vi "sensorTestOutput.vi"() -> ()   [LabVIEW 2018]
panel:
  out "max":dbl
  out "driveAvgFt/s":dbl
  in  "Reset Encoder (Make sure false)":bool
  out "Bound Angle":dbl
  out "climbPoweredIRLeft":bool
  out "climbSkidIRRight":bool
  out "climbPoweredIRRight":bool
  out "lineIRFrontLeft":bool
  out "lineIRFrontRight":bool
  out "lineIRRearLeft":bool
  out "climbSkidIRLeft":bool
  out "cargoYellowIRCVal":bool
  out "lineIRRearRight":bool
  out "driveLeftPositionInch":dbl
  out "driveRightPositionInch":dbl
  out "Button_Y(3)":bool
  out "Button_X(0)":bool
  out "Button_Start(9)":bool
  out "Button_RT(7)":bool
  out "Button_RB(5)":bool
  out "Button_LT(6)":bool
  out "Button_LB(4)":bool
  out "Button_D_Pad_Up(0)":bool
  out "Button_D_Pad_Right(90)":bool
  out "Button_D_Pad_Left(270)":bool
  out "Button_D_Pad_Down(180)":bool
  out "Button_Back(8)":bool
  out "Button_B(2)":bool
  out "Button_A(1)":bool
  out "Axis_Right_Y(3)":dbl
  out "Axis_Right_X(2)":dbl
  out "Axis_Left_Y(1)":dbl
  out "Axis_Left_X(0)":dbl
  out "pitchWind":dbl
  out "yawWind":dbl
  out "driveRightEncoderPosition":i32
  out "driveLeftEncoderPosition":i32
  out "driveIMUYawPitchRoll":cluster{"Yaw":dbl, "Pitch":dbl, "Roll":dbl}
  out "driveFusedHeading":T1
  out "climbRearPosition":i32
  out "climbFrontPosition":i32
  out "rollwind":dbl
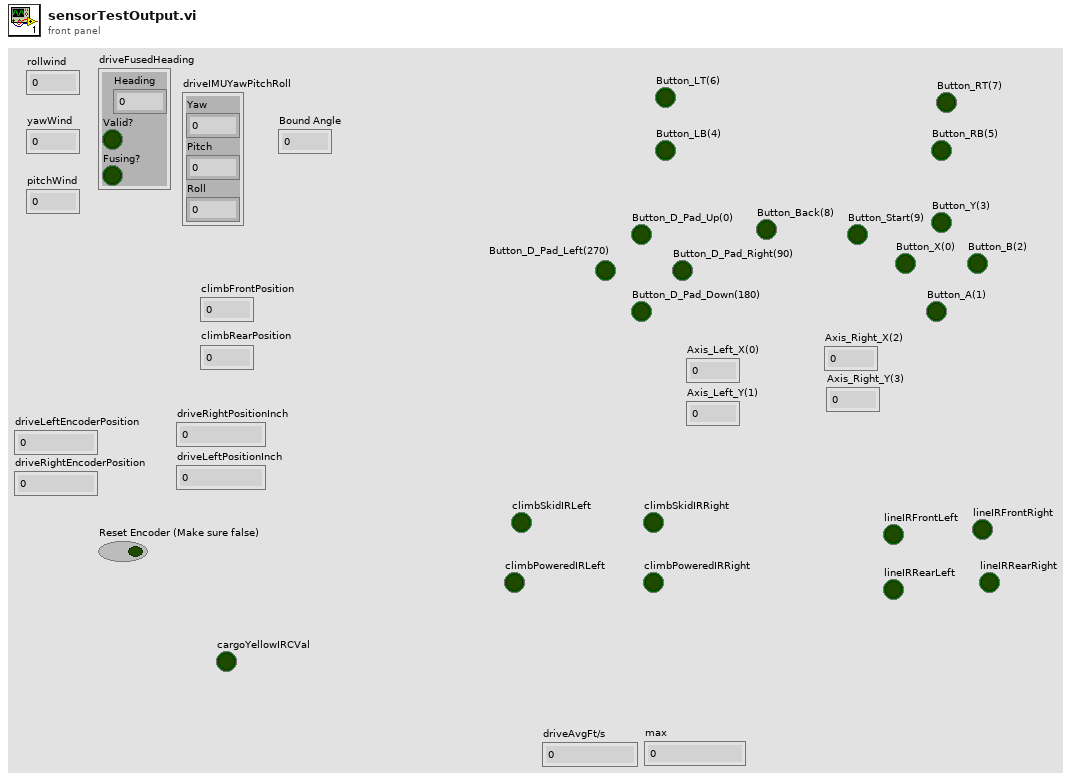
[diagram p1: front panel]
types:
  T1 = cluster{"Heading":dbl, "Valid?":bool, "Fusing?":bool}
  T2 = enum16{"[0, 360]", "[-180, 180]", "[0, 2PI]", "[-PI, PI]"}
  T3 = typedef "WPI_MotorControlDeviceRef.ctl" = cluster{"DeviceStatus":errorcluster, "Type":T4, "PWM":cluster{"PWM Channel":T5, "DeadBand":T6}, "CAN":cluster{"Device Number":u8, "SetOutput VI Ref":variant, "GetOutput VI Ref":variant, "Enable VI Ref":variant, "Disable VI Ref":variant, "Data":variant}, "Invert":bool, "DIO PWM":cluster{"PWM \"Enable\" Channel":T5, "DIOChannel":T7, "PWM Rate":dbl}}
  T4 = typedef "WPI_MotorControlType.ctl" = enum16{"PWM", "CAN", "DIO PWM"}
  T5 = typedef "FPGA_DIOPWMChannel.ctl" = enum8{"PWM 0", "PWM 1", "PWM 2", "PWM 3", "PWM 4", "PWM 5", "PWM 6", "PWM 7", "PWM 8", "PWM 9", "PWM MXP 0", "PWM MXP 1", "PWM MXP 2", "PWM MXP 3", "PWM MXP 4", "PWM MXP 5", "PWM MXP 6", "PWM MXP 7", "PWM MXP 8", "PWM MXP 9", "Invalid"}
  T6 = typedef "WPI_PWMDeadband.ctl" = cluster{"Name":string, "maxPositivePwm":i32, "minPositivePwm":i32, "centerPwm":i32, "maxNegativePwm":i32, "minNegativePwm":i32, "angularRange":u16}
  T7 = typedef "FPGA_DIOChannel.ctl" = enum8{"DIO 0", "DIO 1", "DIO 2", "DIO 3", "DIO 4", "DIO 5", "DIO 6", "DIO 7", "DIO 8", "DIO 9", "DIO MXP 0", "DIO MXP 1", "DIO MXP 2", "DIO MXP 3", "DIO MXP 4", "DIO MXP 5", "DIO MXP 6", "DIO MXP 7", "DIO MXP 8", "DIO MXP 9", "DIO MXP 10", "DIO MXP 11", "DIO MXP 12", "DIO MXP 13", "DIO MXP 14", "DIO MXP 15", "SPI Port CS1", "SPI Port CS2", "SPI Port CS3", "SPI Port MISO", "SPI Port MOSI", "Invalid"}
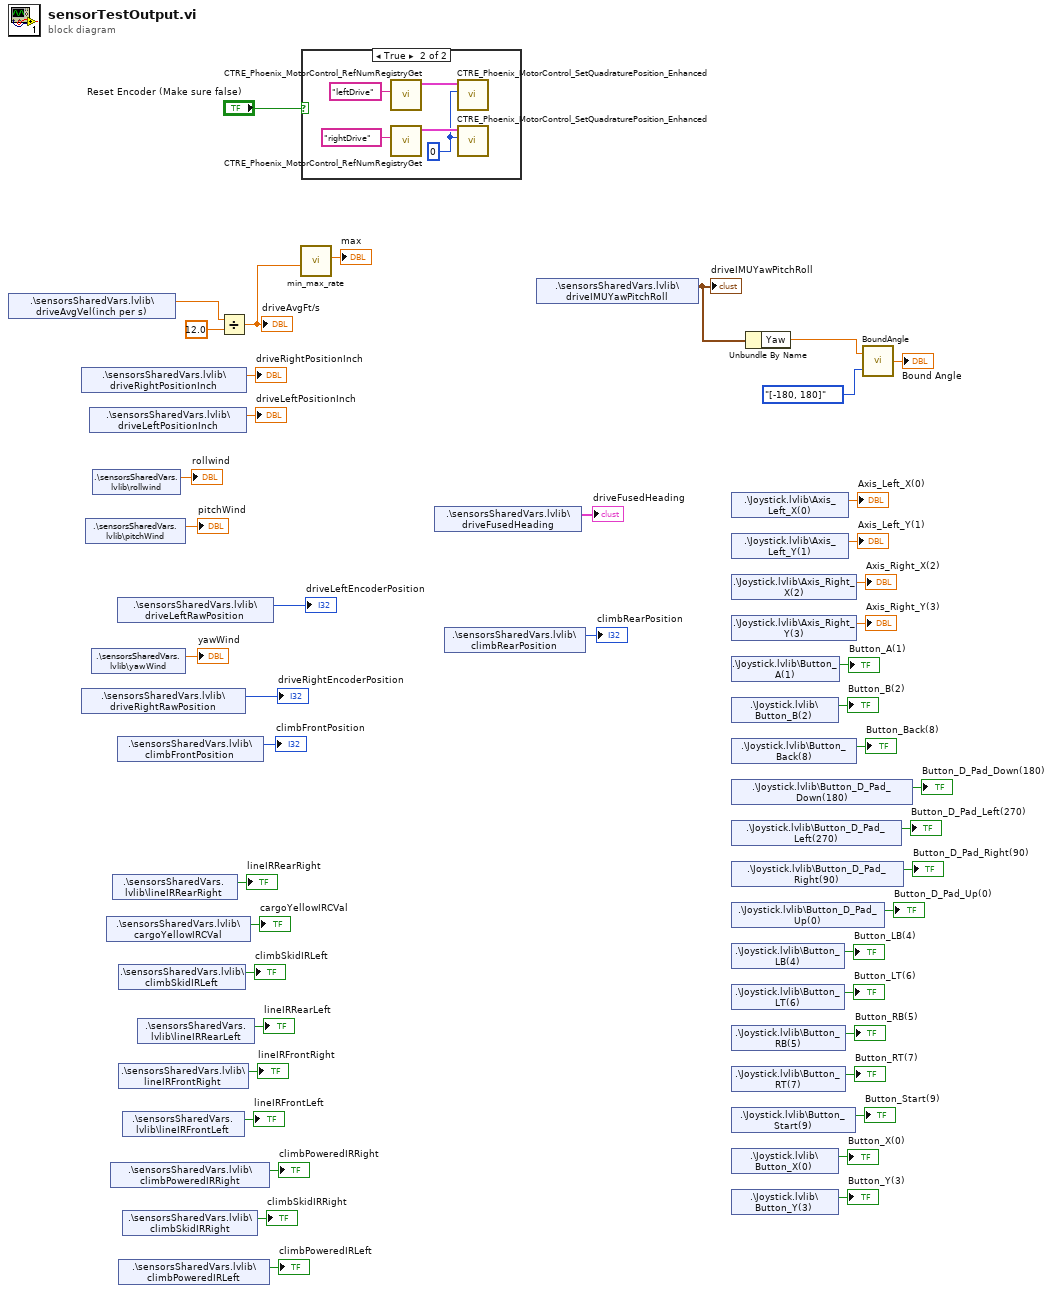
[diagram p0: block diagram]
diagram:
  n1 = shared-variable ".\\sensorsSharedVars.lvlib\\driveAvgVel(inch per s)"() -> (w4:dbl)  [unwired: 1 in, 1 out]
  n2 = shared-variable ".\\sensorsSharedVars.lvlib\\driveRightPositionInch"() -> (→"driveRightPositionInch":dbl)  [unwired: 1 in, 1 out]
  n3 = shared-variable ".\\sensorsSharedVars.lvlib\\driveRightRawPosition"() -> (→"driveRightEncoderPosition":i32)  [unwired: 1 in, 1 out]
  n4 = shared-variable ".\\sensorsSharedVars.lvlib\\pitchWind"() -> (→"pitchWind":dbl)  [unwired: 1 in, 1 out]
  n5 = shared-variable ".\\sensorsSharedVars.lvlib\\driveLeftPositionInch"() -> (→"driveLeftPositionInch":dbl)  [unwired: 1 in, 1 out]
  n6 = shared-variable ".\\sensorsSharedVars.lvlib\\yawWind"() -> (→"yawWind":dbl)  [unwired: 1 in, 1 out]
  n7 = shared-variable ".\\sensorsSharedVars.lvlib\\rollwind"() -> (→"rollwind":dbl)  [unwired: 1 in, 1 out]
  n8 = shared-variable ".\\sensorsSharedVars.lvlib\\cargoYellowIRCVal"() -> (→"cargoYellowIRCVal":bool)  [unwired: 1 in, 1 out]
  n9 = shared-variable ".\\sensorsSharedVars.lvlib\\climbPoweredIRRight"() -> (→"climbPoweredIRRight":bool)  [unwired: 1 in, 1 out]
  n10 = shared-variable ".\\sensorsSharedVars.lvlib\\lineIRRearRight"() -> (→"lineIRRearRight":bool)  [unwired: 1 in, 1 out]
  n11 = shared-variable ".\\sensorsSharedVars.lvlib\\driveLeftRawPosition"() -> (→"driveLeftEncoderPosition":i32)  [unwired: 1 in, 1 out]
  n12 = shared-variable ".\\sensorsSharedVars.lvlib\\climbFrontPosition"() -> (→"climbFrontPosition":i32)  [unwired: 1 in, 1 out]
  n13 = shared-variable ".\\sensorsSharedVars.lvlib\\climbSkidIRLeft"() -> (→"climbSkidIRLeft":bool)  [unwired: 1 in, 1 out]
  n14 = shared-variable ".\\sensorsSharedVars.lvlib\\lineIRFrontRight"() -> (→"lineIRFrontRight":bool)  [unwired: 1 in, 1 out]
  n15 = shared-variable ".\\sensorsSharedVars.lvlib\\climbPoweredIRLeft"() -> (→"climbPoweredIRLeft":bool)  [unwired: 1 in, 1 out]
  n16 = shared-variable ".\\sensorsSharedVars.lvlib\\lineIRFrontLeft"() -> (→"lineIRFrontLeft":bool)  [unwired: 1 in, 1 out]
  n17 = shared-variable ".\\sensorsSharedVars.lvlib\\climbSkidIRRight"() -> (→"climbSkidIRRight":bool)  [unwired: 1 in, 1 out]
  n18 = shared-variable ".\\sensorsSharedVars.lvlib\\lineIRRearLeft"() -> (→"lineIRRearLeft":bool)  [unwired: 1 in, 1 out]
  n19 = Divide(x=w4, y=12.0) -> (x/y=w2:dbl)
  "driveAvgFt/s" <- w2
  n20 = call "min_max_rate.vi"("Rate"=w2) -> ("max"=→"max":dbl)  [unwired: 9 in, 1 out]
  n21 = case shown="True" "Reset Encoder (Make sure false)" {
    frame False {
    }
    frame True {
      w47 = 0 ("New Sensor Position")
      n22 = call <vilib>:"CTRE_Phoenix_MotorControl_RefNumRegistryGet.vi"("refnum name"="leftDrive") -> ("PhoenixMotorControlDevRef"=w49:T3)  [unwired: 9 in, 1 out]
      n23 = call <vilib>:"CTRE_Phoenix_MotorControl_RefNumRegistryGet.vi"("refnum name"="rightDrive") -> ("PhoenixMotorControlDevRef"=w48:T3)  [unwired: 9 in, 1 out]
      n24 = call <vilib>:"CTRE_Phoenix_MotorControl_SetQuadraturePosition_Enhanced.vi"("New Position"=w47, "PhoenixMotorControlDevRef"=w49) -> ()  [unwired: 8 in, 2 out]
      n25 = call <vilib>:"CTRE_Phoenix_MotorControl_SetQuadraturePosition_Enhanced.vi"("New Position"=w47, "PhoenixMotorControlDevRef"=w48) -> ()  [unwired: 8 in, 2 out]
    }
  }
  n26 = shared-variable ".\\sensorsSharedVars.lvlib\\driveFusedHeading"() -> (→"driveFusedHeading":T1)  [unwired: 1 in, 1 out]
  n27 = shared-variable ".\\sensorsSharedVars.lvlib\\climbRearPosition"() -> (→"climbRearPosition":i32)  [unwired: 1 in, 1 out]
  n28 = shared-variable ".\\sensorsSharedVars.lvlib\\driveIMUYawPitchRoll"() -> (w9:cluster{"Yaw":dbl, "Pitch":dbl, "Roll":dbl})  [unwired: 1 in, 1 out]
  "driveIMUYawPitchRoll" <- w9
  n29 = shared-variable ".\\Joystick.lvlib\\Axis_Left_X(0)"() -> (→"Axis_Left_X(0)":dbl)  [unwired: 1 in, 1 out]
  n30 = shared-variable ".\\Joystick.lvlib\\Axis_Left_Y(1)"() -> (→"Axis_Left_Y(1)":dbl)  [unwired: 1 in, 1 out]
  n31 = shared-variable ".\\Joystick.lvlib\\Axis_Right_X(2)"() -> (→"Axis_Right_X(2)":dbl)  [unwired: 1 in, 1 out]
  n32 = shared-variable ".\\Joystick.lvlib\\Axis_Right_Y(3)"() -> (→"Axis_Right_Y(3)":dbl)  [unwired: 1 in, 1 out]
  n33 = shared-variable ".\\Joystick.lvlib\\Button_A(1)"() -> (→"Button_A(1)":bool)  [unwired: 1 in, 1 out]
  n34 = shared-variable ".\\Joystick.lvlib\\Button_B(2)"() -> (→"Button_B(2)":bool)  [unwired: 1 in, 1 out]
  n35 = shared-variable ".\\Joystick.lvlib\\Button_Back(8)"() -> (→"Button_Back(8)":bool)  [unwired: 1 in, 1 out]
  n36 = shared-variable ".\\Joystick.lvlib\\Button_D_Pad_Down(180)"() -> (→"Button_D_Pad_Down(180)":bool)  [unwired: 1 in, 1 out]
  n37 = shared-variable ".\\Joystick.lvlib\\Button_D_Pad_Left(270)"() -> (→"Button_D_Pad_Left(270)":bool)  [unwired: 1 in, 1 out]
  n38 = shared-variable ".\\Joystick.lvlib\\Button_D_Pad_Right(90)"() -> (→"Button_D_Pad_Right(90)":bool)  [unwired: 1 in, 1 out]
  n39 = shared-variable ".\\Joystick.lvlib\\Button_D_Pad_Up(0)"() -> (→"Button_D_Pad_Up(0)":bool)  [unwired: 1 in, 1 out]
  n40 = shared-variable ".\\Joystick.lvlib\\Button_LB(4)"() -> (→"Button_LB(4)":bool)  [unwired: 1 in, 1 out]
  n41 = shared-variable ".\\Joystick.lvlib\\Button_LT(6)"() -> (→"Button_LT(6)":bool)  [unwired: 1 in, 1 out]
  n42 = shared-variable ".\\Joystick.lvlib\\Button_RB(5)"() -> (→"Button_RB(5)":bool)  [unwired: 1 in, 1 out]
  n43 = shared-variable ".\\Joystick.lvlib\\Button_RT(7)"() -> (→"Button_RT(7)":bool)  [unwired: 1 in, 1 out]
  n44 = shared-variable ".\\Joystick.lvlib\\Button_Start(9)"() -> (→"Button_Start(9)":bool)  [unwired: 1 in, 1 out]
  n45 = shared-variable ".\\Joystick.lvlib\\Button_X(0)"() -> (→"Button_X(0)":bool)  [unwired: 1 in, 1 out]
  n46 = shared-variable ".\\Joystick.lvlib\\Button_Y(3)"() -> (→"Button_Y(3)":bool)  [unwired: 1 in, 1 out]
  n47 = Unbundle By Name(w9) -> ("Yaw"=w7:dbl)
  n48 = call <userlib>:"BoundAngle.vi"("Type"=T2."[-180, 180]", "Angle"=w7) -> ("Bound Angle"=→"Bound Angle":dbl)
